vi "Read derived.vi"(8 "error in":errorcluster, 11 "PAS Cell Data in":refnum<class "PAS Cell Data.lvclass">) -> (0 "error out":errorcluster, 2 "derived":T1 {"ext" format="%#.2f"; "noiseLim" format="%#.2g"; "Q" format="%#.2g"}, 3 "PAS Cell Data out":refnum<class "PAS Cell Data.lvclass">)   [LabVIEW 2014, in "PAS Library.lvlib" / "PAS Cell Data.lvclass"]
uses:
  PAS Cell Data.lvclass
  PAS Cell Data.lvclass/PAS Cell Data.ctl
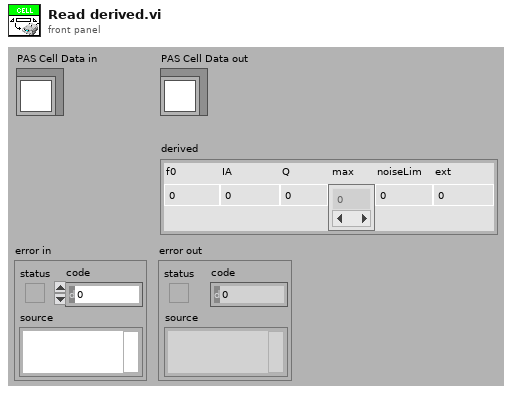
[diagram p1: front panel]
types:
  T1 = cluster{"f0":sgl, "IA":sgl, "Q":sgl, "max":dbl[], "noiseLim":dbl, "ext":dbl}
  T2 = cluster{"f0":sgl, "IA":sgl, "Q":sgl, "max":dbl[], "noiseLim":dbl, "abs":dbl}
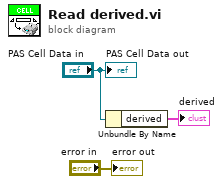
[diagram p0: block diagram]
diagram:
  n1 = Unbundle By Name("PAS Cell Data in") -> ("derived"=→"derived":T2)
  "error out" <- "error in"
  "PAS Cell Data out" <- "PAS Cell Data in"
